vi "SubVI_ReadTDMs Header.vi"(8 "error in":errorcluster, 11 "file path (use dialog)":path=path "D:/Desktop/A  2013-0104-1030-14.txt") -> (0 "error out":errorcluster, 1 "StopTime":dbl, 2 "StartTime":dbl, 3 "tdms file out":refnum<k34>, 4 "Group&ChName":cluster{"Group":string, "ChName":string[]}[](array[cluster]))   [LabVIEW 2012]
panel:
  in  "DataName":cluster{"Group":string, "ChName":string[]}
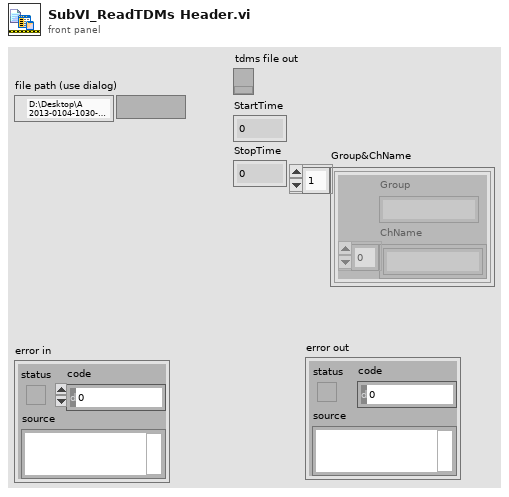
[diagram p1: front panel]
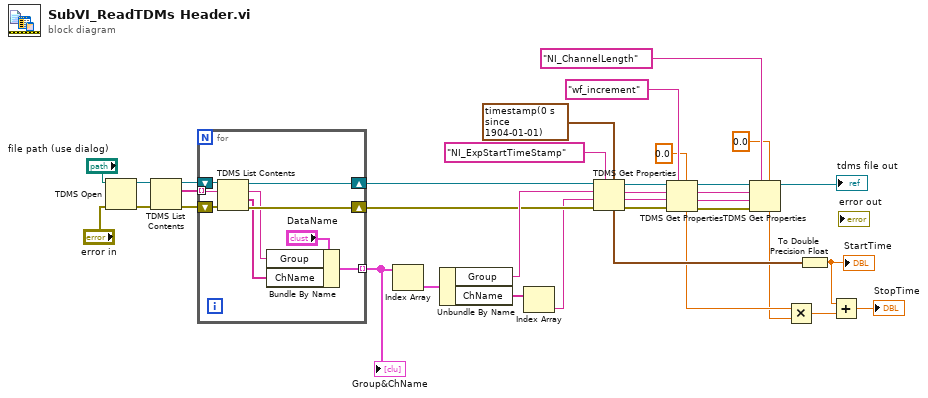
[diagram p0: block diagram]
diagram:
  n1 = TDMS Open(8:"error in", 11:"file path (use dialog)") -> (0:w30:errorcluster, 3:w31:refnum<k34>)  [unwired: 4 in]
  n2 = TDMS List Contents(4:w30, 7:w31) -> (0:w32:errorcluster, 2:w29:string[], 3:w33:refnum<k34>)  [unwired: 1 in, 1 out]
  n3 = for {
    shift-right: [w42] -> w28
    shift-left: w33 -> [w44]
    shift-right: [w41] -> w23
    shift-left: w32 -> [w43]
    tunnel: w29 -> [w39] mode=indexing
    tunnel: [w37] -> w27 mode=indexing
    n4 = TDMS List Contents(4:w43, 6:w39, 7:w44) -> (0:w41:errorcluster, 1:w38:string[], 2:w36:string, 3:w42:refnum<k34>)
    n5 = Bundle By Name(cluster="DataName", "Group"=w36, "ChName"=w38) -> (w37:cluster{"Group":string, "ChName":string[]})
  }
  "Group&ChName" <- w27
  n6 = Index Array(array=w27) -> (element=w26:cluster{"Group":string, "ChName":string[]})  [unwired: 1 in]
  n7 = Unbundle By Name(w26) -> ("Group"=w25:string, "ChName"=w24:string[])
  n8 = Index Array(array=w24) -> (element=w22:string)  [unwired: 1 in]
  n9 = TDMS Get Properties(5:timestamp(0 s since 1904-01-01), 7:"NI_ExpStartTimeStamp" ("属性名称"), 8:w23, 9:w22, 10:w25, 11:w28) -> (0:w18:errorcluster, 1:w8:string, 2:w9:string, 3:w17:refnum<k34>, 4:w19:timestamp)  [unwired: 1 out]
  n10 = TDMS Get Properties(5:0.0, 7:"wf_increment" ("属性名称"), 8:w18, 9:w8, 10:w9, 11:w17) -> (0:w15:errorcluster, 1:w6:string, 2:w7:string, 3:w14:refnum<k34>, 4:w5:dbl)  [unwired: 1 out]
  n11 = TDMS Get Properties(5:0.0, 7:"NI_ChannelLength" ("属性名称"), 8:w15, 9:w6, 10:w7, 11:w14) -> (3:→"tdms file out":refnum<k34>, 4:w4:dbl)  [unwired: 4 out]
  n12 = Multiply(x=w5, y=w4) -> (x*y=w2:dbl)
  n13 = To Double Precision Float(number=w19) -> (double precision float=w3:dbl)
  "StartTime" <- w3
  n14 = Add(x=w3, y=w2) -> (x+y=→"StopTime":dbl)
